vi "LDO_Setup_Parameters.vi"(0 "UI in":refnum<queue>, 1 "Modbus":refnum<queue>, 2 "Initialize?":bool, 3 "Alicat_GasMeter":refnum<queue>, 5 "Vesta LDO":refnum<queue>, 9 "Vesta ON Temperature (LDO)":T1={"Water Heater Temp (°F)"=135, "Differential  (°F)"=10.0} {"Water Heater Temp (°F)" min=32 max=203}, 11 "error in (no error)":errorcluster) -> (15 "error out":errorcluster)   [LabVIEW 2020]
uses:
  Message Queue/Message Cluster.ctl
  Drivers/Resideo Gas Valve/Type Definitions/Temperature Control.ctl
  Message Queue/Enqueue Message (Single).vi
  Message Queue/Message Queue.lvlib
panel:
  out "UI Output":refnum<queue>
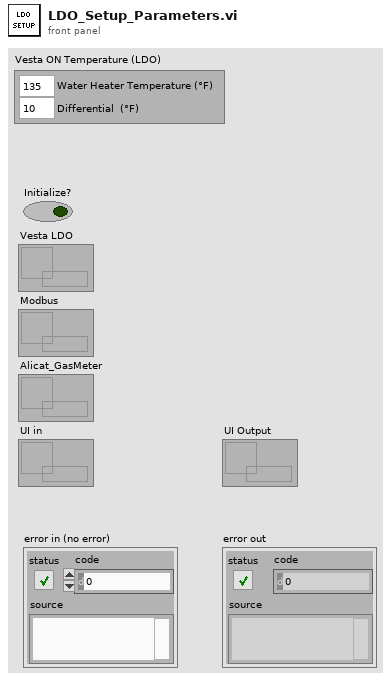
[diagram p1: front panel]
types:
  T1 = typedef "Temperature Control.ctl" = cluster{"Water Heater Temp (°F)":u16, "Differential  (°F)":dbl}
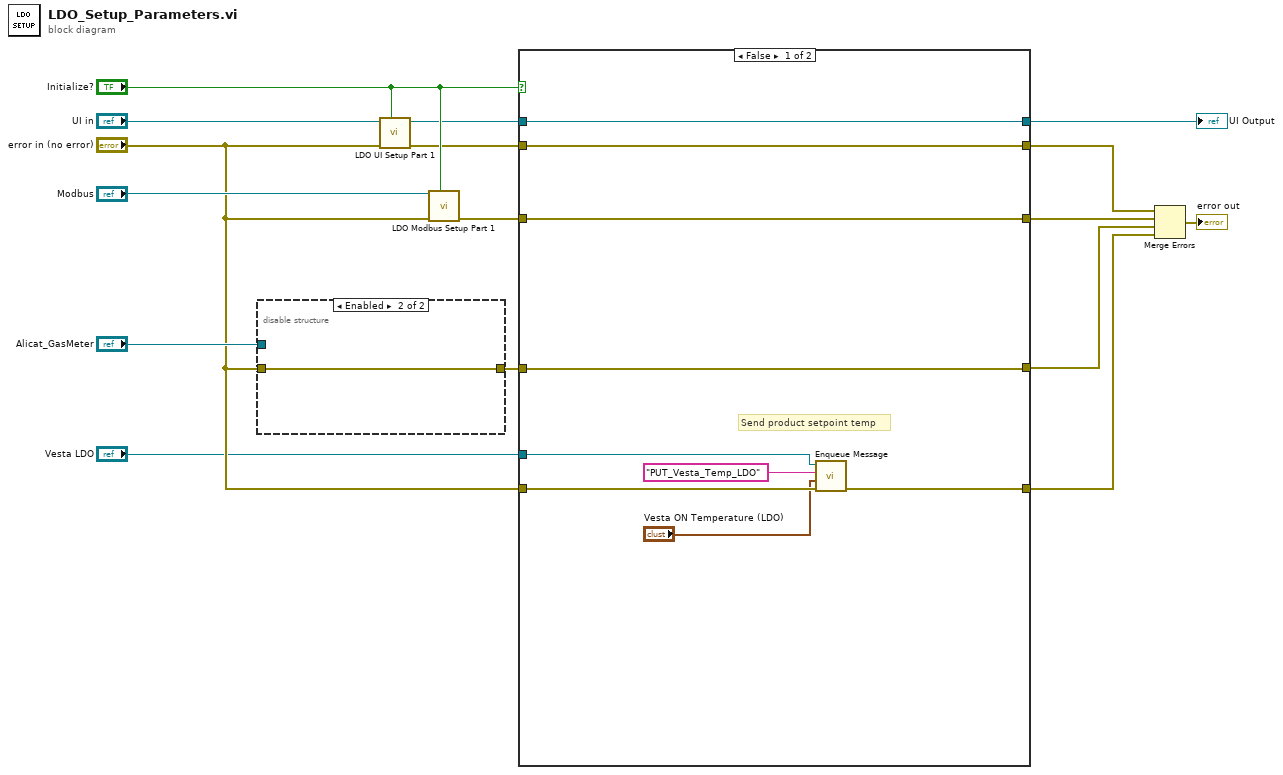
[diagram p0: block diagram]
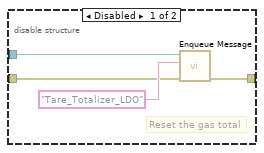
[diagram p2: hidden frame]
diagram:
  n1 = disable-structure shown="Enabled" {
    disable-tunnel: "Alicat_GasMeter" -> [w19 _]
    disable-tunnel: [w18 w21] -> w10
    disable-tunnel: "error in (no error)" -> [w17 w21]
    frame Disabled {
      # "Reset the gas total"
      n2 = call-poly "Enqueue Message.vi"("error in (no error)"=w17, "Message"="Tare_Totalizer_LDO", "Message Queue"=w19) -> ("error out"=w18:errorcluster)  [unwired: 7 in, 1 out]
    }
    frame Enabled {
    }
  }
  n3 = call "LDO UI Setup Part 1.vi"("Initialize? in"="Initialize?", "error in (no error)"="error in (no error)", "Queue in"="UI in") -> ("error out"=w12:errorcluster, "dup Message Queue"=w3:refnum<queue>)  [unwired: 7 in]
  n4 = call "LDO Modbus Setup Part 1.vi"("Initialize?"="Initialize?", "error in (no error)"="error in (no error)", "Queue in"="Modbus") -> ("error out"=w11:errorcluster)  [unwired: 7 in, 1 out]
  n5 = case shown="False" "Initialize?" {
    tunnel: w12 -> [w30 w32]
    tunnel: [w30 w32] -> w8
    tunnel: w11 -> [w29 w33]
    tunnel: [w29 w33] -> w7
    tunnel: w10 -> [w28 w34]
    tunnel: [w28 w34] -> w6
    tunnel: "error in (no error)" -> [w25 w35]
    tunnel: [w24 w35] -> w5
    tunnel: w3 -> [w27 w31]
    tunnel: [w27 w31] -> w2
    tunnel: "Vesta LDO" -> [w23 _]
    frame False {
      # "Send product setpoint temp"
      n6 = call-poly "Enqueue Message.vi"("error in (no error)"=w25, "Message Data"="Vesta ON Temperature (LDO)", "Message"="PUT_Vesta_Temp_LDO", "Message Queue"=w23) -> ("error out"=w24:errorcluster)  [unwired: 6 in, 1 out]
    }
    frame True {
    }
  }
  "UI Output" <- w2
  n7 = Merge Errors(w8, w7, w6, w5) -> (→"error out":errorcluster)
